vi "updateDest.vi"(8 "error in (no error)":errorcluster, 10 "NewAllyRobots":refnum<class "Robot.lvclass">[](array[class]), 11 "LastAlly":refnum<class "Ally.lvclass">) -> (0 "error out":errorcluster, 2 "NewAllyRobotsUpdated":refnum<class "Robot.lvclass">[](array[class]), 3 "Ally out":refnum<class "Ally.lvclass">)   [LabVIEW 2023, in "Ally.lvclass"]
uses:
  Ally.lvclass
  C:/Users/lucio/Desktop/roboime/SSL_AI/Team_class/Team.lvclass
  Robot_class/Robot.lvclass
  Team_class/Team.lvclass/Team.ctl
  Robot_class/Robot.lvclass/Robot.ctl
  Robot_class/Write kick_x.vi
  Robot_class/Write kick_z.vi
  Robot_class/Write dest_x.vi
  Robot_class/Write dest_y.vi
  Robot_class/Write dest_orientation.vi
  Robot_class/Write dest_x_kick.vi
  Robot_class/Write dest_y_kick.vi
  Robot_class/Write tactic.vi
  Robot_class/Read id.vi
  Robot_class/Read kick_x.vi
  Robot_class/Read kick_z.vi
  Robot_class/Read dest_x.vi
  Robot_class/Read dest_y.vi
  Robot_class/Read dest_orientation.vi
  Robot_class/Read dest_x_kick.vi
  Robot_class/Read dest_y_kick.vi
  Robot_class/Read tactic.vi
  Robot_class/Read keepDest.vi
  Team_class/Read RobotRef.vi
  Utilities_class/Utilities.lvclass
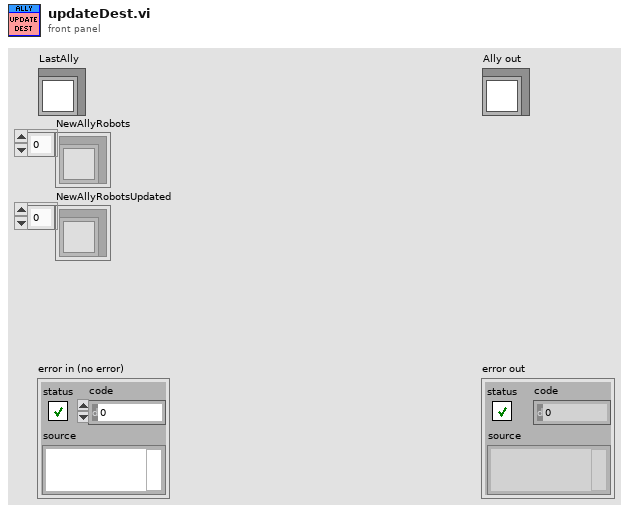
[diagram p1: front panel]
types:
  T1 = typedef "tactics.ctl" = enum16{"GoToBallPlacementPosition", "PlaceBall", "GoToBallPlacement", "5Robots", "BallPlacementEnemy", "ReceivePassInFuturePoint", "Roller", "PrepareRollToPassRollerGoTo", "PrepareRollToPassReceiverGoTo", "WaitRoll", "PositionToRoll", "PenaltyAttacker", "PassObserver", "PenaltyDefense", "TableReceiverTactic", "Test", "DefendGoal", "Marker", "FollowAttacker", "DefendArea", "Shoot", "AttackerAimGoal", "AttackerBallOutOfField", "AttackerBlock", "AttackerStop", "Duelist", "Halt", "ZigZag", "GoTo", "Timeout", "KickToBestRobot", "KickToPassReceiver", "PositionToReceivePass", "WaitPass", "GoToTarget"}
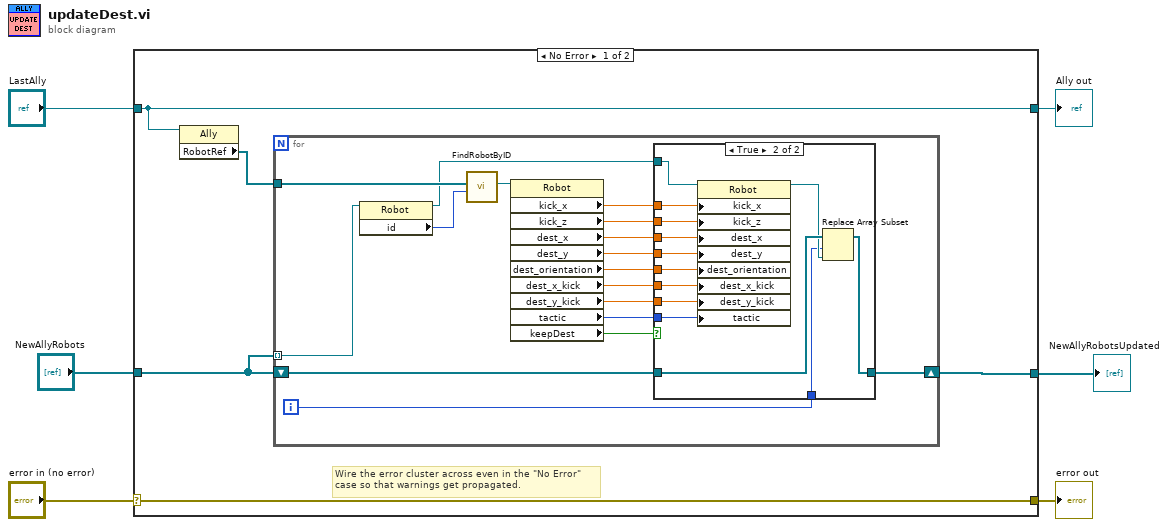
[diagram p0: block diagram]
diagram:
  n1 = case shown="No Error" "error in (no error)" {
    selector: "error in (no error)" -> [w11 w44]
    tunnel: [w11 w44] -> w5
    tunnel: [w10 w43] -> w3
    tunnel: "LastAlly" -> [w10 w43]
    tunnel: "NewAllyRobots" -> [w7 _]
    tunnel: [w8 _] -> w1
    frame No Error {
      # "Wire the error cluster across even in the \"No Error\"\ncase so that warnings get propagated."
      n2 = property class="Ally"(reference=w10) -> ("RobotRef"=w9:refnum<class "Robot.lvclass">[])  [unwired: 1 in, 2 out]
      n3 = for {
        tunnel: w9 -> [w26]
        shift-right: [w14] -> w8
        shift-left: w7 -> [w16]
        tunnel: w7 -> [w28] mode=indexing
        i -> [w15]
        n4 = property class="Robot"(reference=w28) -> (reference out=w23:refnum<class "Robot.lvclass">, "id"=w27:i32)  [unwired: 1 in, 1 out]
        n5 = call "FindRobotByID.vi"("id"=w27, "RobotRef"=w26) -> ("Robot"=w25:refnum<class "Robot.lvclass">)  [unwired: 6 in, 3 out]
        n6 = property class="Robot"(reference=w25) -> ("kick_x"=w13:dbl, "kick_z"=w12:dbl, "dest_x"=w22:dbl, "dest_y"=w21:dbl, "dest_orientation"=w20:dbl, "dest_x_kick"=w19:dbl, "dest_y_kick"=w18:dbl, "tactic"=w17:T1, "keepDest"=w24:bool)  [unwired: 1 in, 2 out]
        n7 = case shown="True" w24 {
          tunnel: w23 -> [_ w42]
          tunnel: w22 -> [_ w41]
          tunnel: w21 -> [_ w40]
          tunnel: w20 -> [_ w39]
          tunnel: w19 -> [_ w38]
          tunnel: w18 -> [_ w37]
          tunnel: w17 -> [_ w36]
          tunnel: w16 -> [w29 w35]
          tunnel: w15 -> [_ w33]
          tunnel: [w29 w32] -> w14
          tunnel: w13 -> [_ w31]
          tunnel: w12 -> [_ w30]
          frame False {
          }
          frame True {
            n8 = property class="Robot"(reference=w42, "kick_x"=w31, "kick_z"=w30, "dest_x"=w41, "dest_y"=w40, "dest_orientation"=w39, "dest_x_kick"=w38, "dest_y_kick"=w37, "tactic"=w36) -> (reference out=w34:refnum<class "Robot.lvclass">)  [unwired: 1 in, 1 out]
            n9 = Replace Array Subset(array=w35, new element=w34, index=w33) -> (w32:refnum<class "Robot.lvclass">[])
          }
        }
      }
    }
    frame Error {
    }
  }
  "error out" <- w5
  "Ally out" <- w3
  "NewAllyRobotsUpdated" <- w1
